vi "坐标.vi"(0 "线段":cluster{"X":dbl, "Y":dbl, "Z":dbl}[](array[cluster])=[{"X"=1.0, "Y"=1.0, "Z"=1.0}, {"X"=0.0, "Y"=6.0, "Z"=-8.0}, {"X"=9.0, "Y"=7.0, "Z"=2.0}], 1 "刀具坐标":cluster{"X":sgl, "Y":sgl, "Z":sgl}, 2 "坐标和刀具参数":T2={"XYZ轴显示大小"={"Length"=7.0, "Radius"=0.3, "Character Size"=4.3, "坐标颜色"=14679826}, "刀具大小"={"Height"=10.0, "Radius"=2.0, "刀具颜色"=15666944}}, 3 "error in (no error)":errorcluster caption="错误输入（无错误）") -> (7 "Scene Object Out":refnum<vi> caption="场景对象输出", 10 "error out":errorcluster caption="错误输出")   [LabVIEW 2019]
uses:
  <vilib>/Utility/miscctls.llb/LV3DPointTypeDef.ctl
  <vilib>/Utility/miscctls.llb/LVRectTypeDef.ctl
  <vilib>/picture/3D Picture Control/Object/Create Object (drawable).vi
  <vilib>/picture/3D Picture Control/Object/Add Object (no reference).vi
  <vilib>/picture/3D Picture Control/NI_3D Picture Control.lvlib
panel:
  out "项标识符 2":string
  out "项路径 2":string
  out "三维图片":refnum<vi>(3d-picture)
  in  "坐标控件方向":cluster{"视角位置":T1, "对象":T1, "向上方向":T1}={"视角位置"={"X"=0.0, "Y"=0.0, "Z"=-100.0}, "对象"={"X"=0.0, "Y"=0.0, "Z"=0.0}, "向上方向"={"X"=0.0, "Y"=1.0, "Z"=0.0}}
  out "结果":bool
  in  "值":bool
  in  "显示方式":enum16{"Scene Window", "Scene Display"}(ring)=enum."Scene Display"
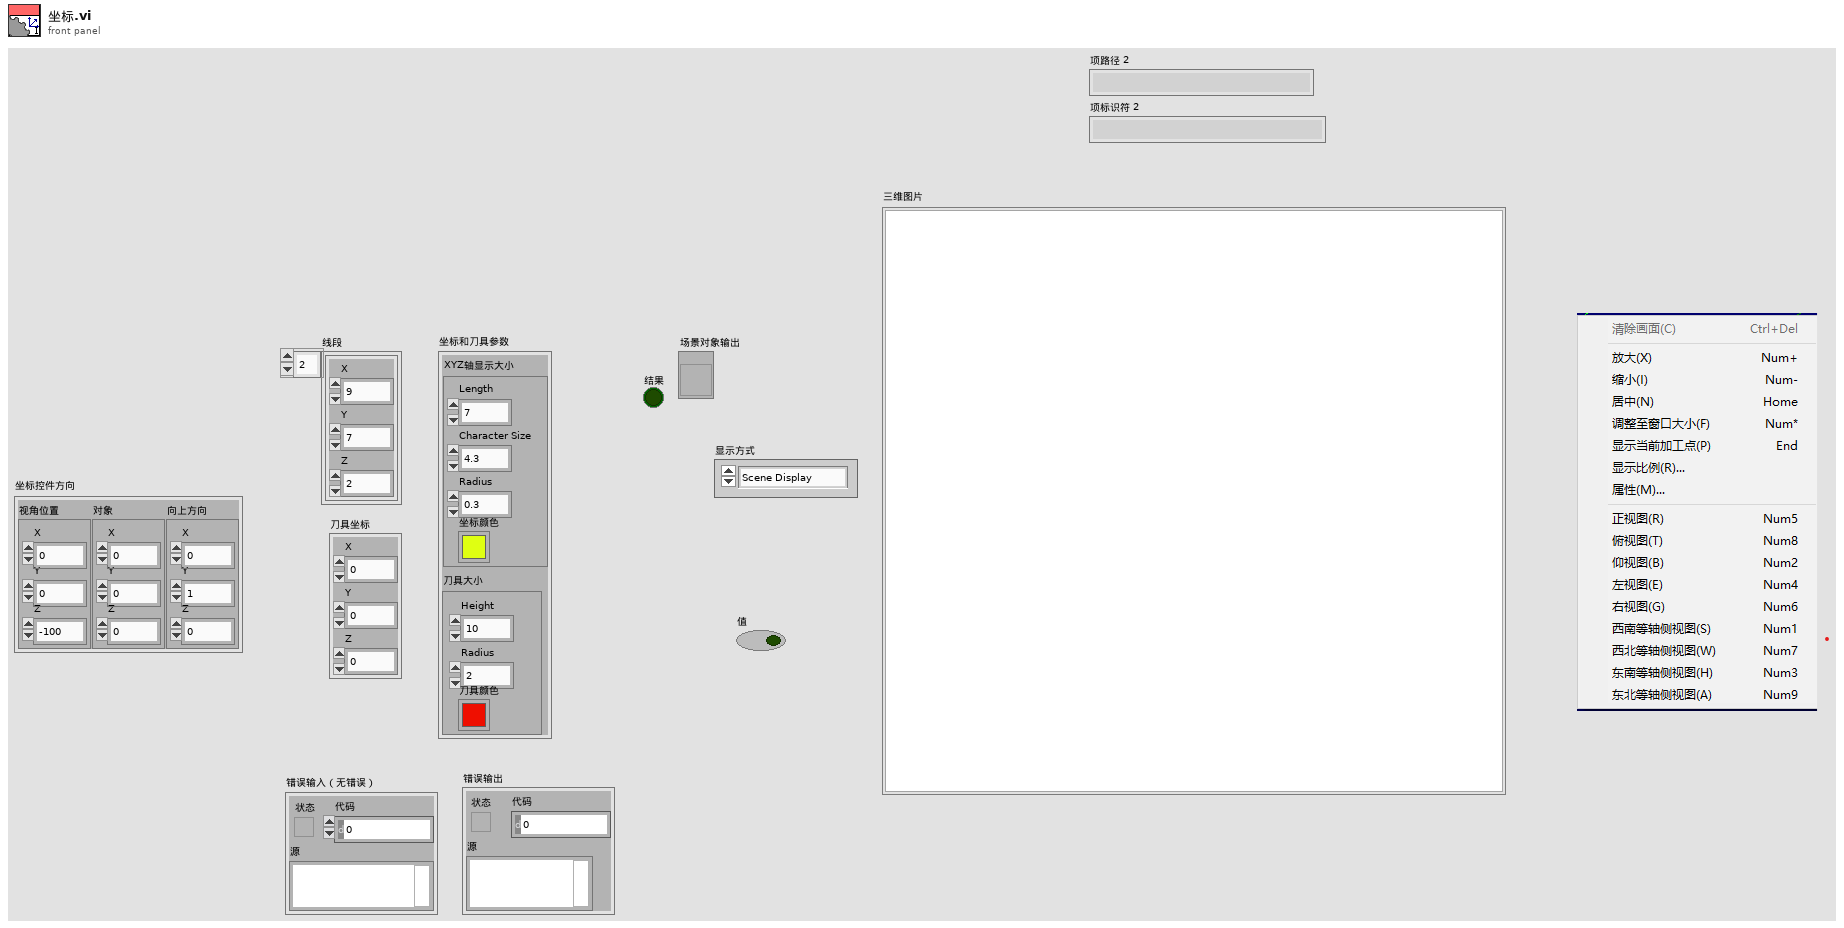
[diagram p1: front panel]
types:
  T1 = typedef "LV3DPointTypeDef.ctl" = cluster{"X":sgl, "Y":sgl, "Z":sgl}
  T2 = cluster{"XYZ轴显示大小":cluster{"Length":sgl, "Radius":sgl, "Character Size":sgl, "坐标颜色":u32}, "刀具大小":cluster{"Height":sgl, "Radius":sgl, "刀具颜色":u32}}
  T3 = enum16{"Overall", "Per Primitive", "Per Vertex", "Binding Off"}
  T4 = enum16{"Inherit Material", "Use entire Material", "Ignore Ambient", "Ignore Diffuse", "Ignore Specular", "Ignore Emission", "Ignore Ambient and Diffuse"}
  T5 = enum16{"None", "Spherical", "Flying", "Oriented"}
  T6 = enum16{"Open", "Minimized", "Maximized", "Hidden"}
  T7 = enum16{"Inherit Value", "Points", "Wireframe", "Polygons"}
  T8 = typedef "LVRectTypeDef.ctl" = cluster{"Left":i16, "Top":i16, "Right":i16, "Bottom":i16}
  T9 = enum16{"Points", "Lines", "Line Strip", "Line Loop", "Triangles", "Triangle Strip", "Triangle Fan", "Quads", "Quad Strip", "Polygon"}
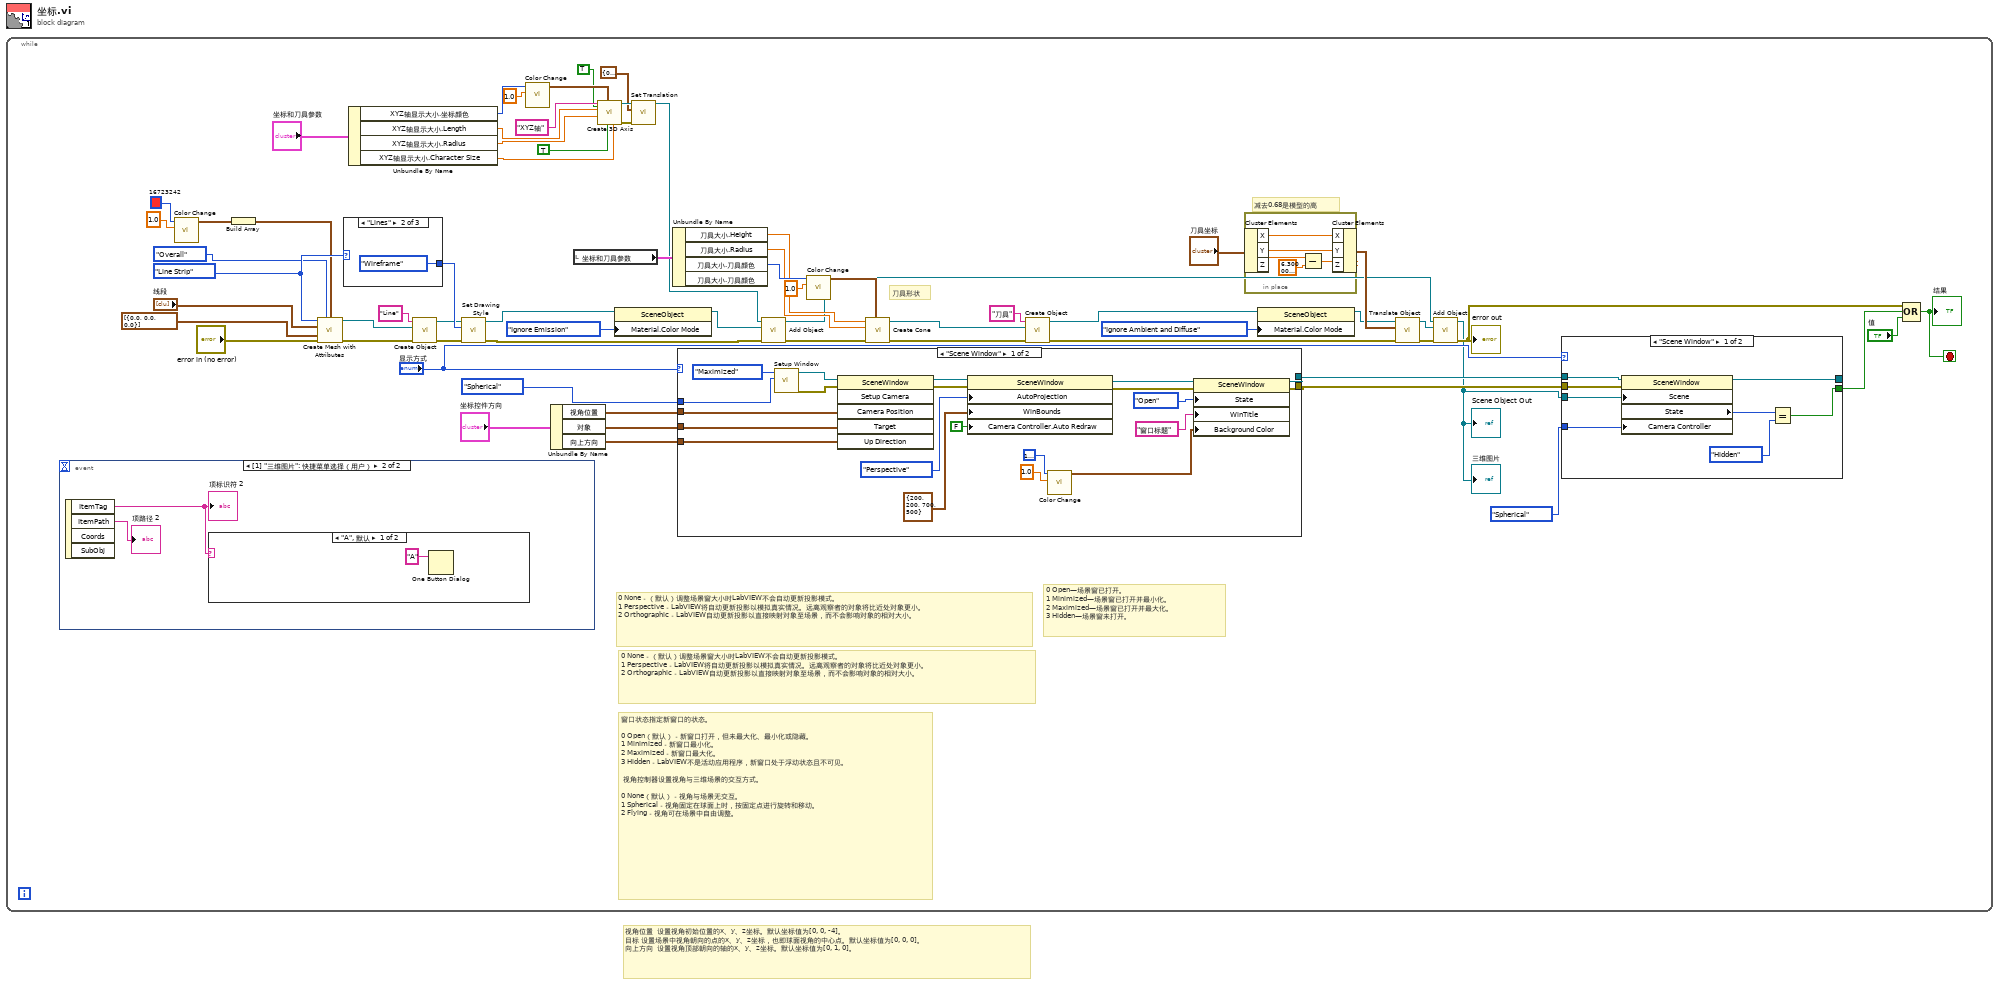
[diagram p0: block diagram]
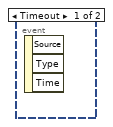
[diagram p2: hidden frame]
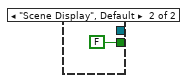
[diagram p4: hidden frame]
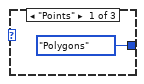
[diagram p5: hidden frame]
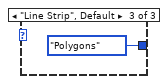
[diagram p6: hidden frame]
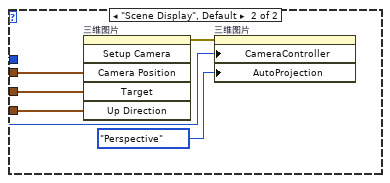
[diagram p7: hidden frame]
diagram:
  # "视角位置  设置视角初始位置的x、y、z坐标。默认坐标值为[0, 0, -4]。 \n目标 设置场景中视角朝向的点的x、y、z坐标，也即球面视角的中心点。默认坐标值为[0, 0, 0]。  \n向上方向  设置视角顶部朝向的轴的x、y、z坐标。默认坐标值为[0, 1, 0]。"
  n1 = while {
    stop <- w1 stop-if-true
    w58 = T9."Line Strip" ("Draw Mode")
    # "减去0.68是模型的高"
    # "刀具形状"
    # "0 None－（默认）调整场景窗大小时LabVIEW不会自动更新投影模式。 \n1 Perspective－LabVIEW将自动更新投影以模拟真实情况。远离观察者的对象将比近处对象更小。 \n2 Orthographic－LabVIEW自动更新投影以直接映射对象至场景，而不会影响对象的相对大小。"
    # "0 Open—场景窗已打开。 \n1 Minimized—场景窗已打开并最小化。 \n2 Maximized—场景窗已打开并最大化。 \n3 Hidden—场景窗未打开。"
    # "0 None－（默认）调整场景窗大小时LabVIEW不会自动更新投影模式。 \n1 Perspective－LabVIEW将自动更新投影以模拟真实情况。远离观察者的对象将比近处对象更小。 \n2 Orthographic－LabVIEW自动更新投影以直接映射对象至场景，而不会影响对象的相对大小。"
    # "窗口状态指定新窗口的状态。 \n\n0 Open（默认）－新窗口打开，但未最大化、最小化或隐藏。 \n1 Minimized－新窗口最小化。 \n2 Maximized－新窗口最大化。 \n3 Hidden－LabVIEW不是活动应用程序，新窗口处于浮动状态且不可见。 \n \n 视角控制器设置视角与三维场景的交互方式。 \n\n0 None（默认）－视角与场景无交互。 \n1 Spherical－视角固定在球面上时，按固定点进行旋转和移动。 \n2 Flying－视角可在场景中自由调整。"
    n2 = event shown="[1] \"三维图片\": 快捷菜单选择（用户）" {
      selector: _ -> [_ _]
      dyn-events: _ -> [_ _]
      timeout: _ -> [_ _]
      event Timeout {
        n3 = event-data() -> ()  [unwired: 1 in, 3 out]
      }
      event "三维图片": Shortcut Menu Selection (User) {
        n4 = event-data() -> ("ItemTag"=w68:string, "ItemPath"=→"项路径 2":string)  [unwired: 1 in, 2 out]
        "项标识符 2" <- w68
        n5 = case shown="\"A\", 默认" w68 {
          frame "A", Default {
            n6 = One Button Dialog(message="A" ("消息")) -> ()  [unwired: 1 in, 1 out]
          }
          frame "Q" {
          }
        }
      }
    }
    n7 = call <vilib>:"Color Change.vi"("Alpha"=1.0, "Color"=u32 16723242) -> ("RGBA"=w54:cluster{"R":sgl, "G":sgl, "B":sgl, "A":sgl})  [unwired: 9 in]
    n8 = Build Array(w54) -> (w53:cluster{"R":sgl, "G":sgl, "B":sgl, "A":sgl}[])
    n9 = call <vilib>:"Create Mesh with Attributes.vi"("Draw Mode"=w58, "Color Binding Mode"=T3."Overall", "Color Array"=w53, "Vertex Array"="线段", "Normal Array"=cluster{"X":sgl, "Y":sgl, "Z":sgl}[] [{"X"=0.0, "Y"=0.0, "Z"=0.0}], "error in (no error)"="error in (no error)") -> ("New Mesh Refnum"=w43:refnum<vi>, "error out"=w52:errorcluster)  [unwired: 8 in]
    n10 = case shown="\"Lines\"" w58 {
      tunnel: [T7."Polygons" ("Mode") T7."Wireframe" ("Mode") T7."Polygons" ("Mode")] -> w57
      frame "Points" {
      }
      frame "Lines" {
      }
      frame "Line Strip", Default {
      }
    }
    n11 = Unbundle By Name("坐标和刀具参数") -> ("XYZ轴显示大小.坐标颜色"=w2:u32, "XYZ轴显示大小.Length"=w23:sgl, "XYZ轴显示大小.Radius"=w22:sgl, "XYZ轴显示大小.Character Size"=w21:sgl)
    n12 = call-poly <vilib>:"Create Object.vi"("error in (no error)"=w52, "Geometry"=w43, "Name"="Line") -> ("error out"=w51:errorcluster, "Scene:New Object"=w41:refnum<vi>)  [unwired: 7 in]
    n13 = call <vilib>:"Set Drawing Style.vi"("error in (no error)"=w51, "Mode"=w57, "Scene Object In"=w41) -> ("error out"=w39:errorcluster, "Scene Object Out"=w11:refnum<vi>)  [unwired: 7 in]
    n14 = call <vilib>:"Color Change.vi"("Alpha"=1.0, "Color"=w2) -> ("RGBA"=w50:cluster{"R":sgl, "G":sgl, "B":sgl, "A":sgl})  [unwired: 9 in]
    n15 = Unbundle By Name("坐标控件方向") -> ("视角位置"=w61:T1, "对象"=w60:T1, "向上方向"=w59:T1)
    n16 = local read "坐标和刀具参数"() -> (w20:T2)
    n17 = call <vilib>:"Create 3D Axis.vi"("Character Size"=w21, "Half plane?"=TRUE, "Axis label?"=TRUE, "Color"=w50, "Radius"=w22, "Length"=w23, "Name"="XYZ轴") -> ("error out"=w45:errorcluster, "New Object Refnum"=w47:refnum<vi>)  [unwired: 3 in]
    n18 = property class="SceneObject"(reference=w11, "Material.Color Mode"=T4."Ignore Emission" ("材质:颜色模式")) -> (reference out=w10:refnum<vi>)  [unwired: 1 in, 1 out]
    n19 = call <vilib>:"Set Translation.vi"("error in (no error)"=w45, "Translation"=cluster{"X":sgl, "Y":sgl, "Z":sgl} {"X"=0.0, "Y"=0.0, "Z"=0.0}, "Scene Object"=w47) -> ("Translated Object"=w12:refnum<vi>)  [unwired: 7 in, 1 out]
    n20 = Unbundle By Name(w20) -> ("刀具大小.Height"=w18:sgl, "刀具大小.Radius"=w17:sgl, "刀具大小.刀具颜色"=w19:u32)  [unwired: 1 out]
    n21 = case shown="\"Scene Window\"" "显示方式" {
      tunnel: enum16{"None", "Spherical", "Flying"}."Spherical" ("Camera Controller") -> [w96 w112]
      tunnel: [w95 _] -> w63
      tunnel: [w94 _] -> w64
      tunnel: w61 -> [w93 w111]
      tunnel: w60 -> [w92 w110]
      tunnel: w59 -> [w87 w109]
      frame "Scene Window" {
        n22 = call <vilib>:"Setup Window.vi"("Camera Controller"=w96, "Window State"=T6."Maximized") -> ("error out"=w99:errorcluster, "New Window Refnum"=w98:refnum<vi>)  [unwired: 8 in]
        n23 = invoke class="SceneWindow" method="Setup Camera"(reference=w98, error in=w99, "Camera Position"=w93, "Target"=w92, "Up Direction"=w87) -> (reference out=w107:refnum<vi>, error out=w106:errorcluster)  [unwired: 1 in, 4 out]
        n24 = property on="属性节点" class="SceneWindow"(reference=w107, error in=w106, "AutoProjection"=enum16{"None", "Perspective", "Orthographic"}."Perspective" ("自动投影模式"), "WinBounds"=T8 {"Left"=200, "Top"=200, "Right"=700, "Bottom"=500} ("窗口边界"), "Camera Controller.Auto Redraw"=FALSE ("视角控制器:自动重绘")) -> (reference out=w104:refnum<vi>, error out=w105:errorcluster)
        n25 = call <vilib>:"Color Change.vi"("Alpha"=1.0, "Color"=u32 16777216) -> ("RGBA"=w88:cluster{"R":sgl, "G":sgl, "B":sgl, "A":sgl})  [unwired: 9 in]
        n26 = property class="SceneWindow"(reference=w104, error in=w105, "State"=T6."Open" ("窗口状态"), "WinTitle"="窗口标题" ("窗口标题"), "Background Color"=w88) -> (reference out=w95:refnum<vi>, error out=w94:errorcluster)
      }
      frame "Scene Display", Default {
        n27 = invoke on="三维图片" class="SceneGraphDisp (严格)" method="Setup Camera"("Camera Position"=w111, "Target"=w110, "Up Direction"=w109) -> (error out=w108:errorcluster)  [unwired: 3 in, 5 out]
        n28 = property on="三维图片" class="SceneGraphDisp (严格)"(error in=w108, "CameraController"=w112, "AutoProjection"=enum16{"None", "Perspective", "Orthographic"}."Perspective" ("自动投影模式")) -> ()  [unwired: 1 in, 2 out]
      }
    }
    n29 = call-poly <vilib>:"Add Object.vi"("error in (no error)"=w39, "New Object In"=w10, "Scene Object In"=w12) -> ("error out"=w4:errorcluster, "Scene Object Out"=w5:refnum<vi>)  [unwired: 7 in]
    n30 = call <vilib>:"Color Change.vi"("Alpha"=1.0, "Color"=w19) -> ("RGBA"=w36:cluster{"R":sgl, "G":sgl, "B":sgl, "A":sgl})  [unwired: 9 in]
    n31 = call <vilib>:"Create Cone.vi"("Color"=w36, "error in (no error)"=w4, "Radius"=w17, "Height"=w18) -> ("error out"=w35:errorcluster, "New Cone Refnum"=w38:refnum<vi>)  [unwired: 6 in]
    n32 = call-poly <vilib>:"Create Object.vi"("error in (no error)"=w35, "Geometry"=w38, "Name"="刀具") -> ("error out"=w31:errorcluster, "Scene:New Object"=w8:refnum<vi>)  [unwired: 7 in]
    n33 = in-place {
      n34 = in-place-cluster #1("刀具坐标") -> ("X"=w83:sgl, "Y"=w82:sgl, "Z"=w81:sgl)
      n35 = Subtract(x=w81, y=sgl 6.3) -> (x-y=w80:sgl)
      n36 = in-place-cluster #1("X"=w83, "Y"=w82, "Z"=w80) -> (w29:cluster{"X":sgl, "Y":sgl, "Z":sgl})
    }
    n37 = property class="SceneObject"(reference=w8, "Material.Color Mode"=T4."Ignore Ambient and Diffuse" ("材质:颜色模式")) -> (reference out=w7:refnum<vi>)  [unwired: 1 in, 1 out]
    n38 = call <vilib>:"Translate Object.vi"("error in (no error)"=w31, "Translation"=w29, "Scene.Object In"=w7) -> ("error out"=w25:errorcluster, "Scene.Object Out"=w30:refnum<vi>)  [unwired: 7 in]
    n39 = call-poly <vilib>:"Add Object.vi"("error in (no error)"=w25, "New Object In"=w30, "Scene Object In"=w5) -> ("error out"=w13:errorcluster, "Scene Object Out"=w3:refnum<vi>)  [unwired: 7 in]
    "error out" <- w13
    "Scene Object Out" <- w3
    "三维图片" <- w3
    n40 = case shown="\"Scene Window\"" "显示方式" {
      tunnel: w3 -> [w77 _]
      tunnel: w64 -> [w76 _]
      tunnel: [w73 FALSE] -> w16
      tunnel: T5."Spherical" ("视角控制器:类型") -> [w72 _]
      tunnel: w63 -> [w71 _]
      tunnel: [w70 _] -> _
      frame "Scene Window" {
        n41 = property class="SceneWindow"(reference=w71, error in=w76, "Scene"=w77, "Camera Controller"=w72) -> (reference out=w70:refnum<vi>, "State"=w75:T6)  [unwired: 1 out]
        n42 = Equal?(x=w75, y=T6."Hidden" ("窗口状态")) -> (x = y?=w73:bool)
      }
      frame "Scene Display", Default {
      }
    }
    n43 = Compound Arithmetic op=OR ("复合运算")(w13, w16, "值") -> (w1:bool)
    "结果" <- w1
  }
